vi "Read OD data.vi"(4 "OD num":dbl) -> (1 "OD data":dbl[][](array[numeric]) caption="所有行" format="%0.3f")   [LabVIEW 2013]
panel:
  out "路径":path
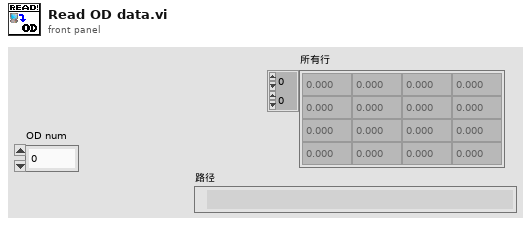
[diagram p1: front panel]
types:
  T1 = typedef "imagedata.ctl" = cluster{"image type":i32, "image depth":i32, "image":u8[], "mask":u8[], "colors":u32[], "Rectangle":cluster{"left":i16, "top":i16, "right":i16, "bottom":i16}}
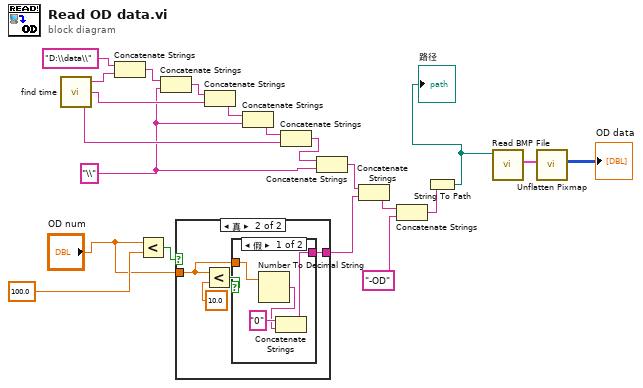
[diagram p0: block diagram]
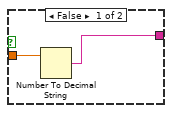
[diagram p2: hidden frame]
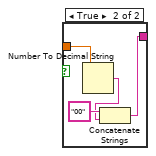
[diagram p3: hidden frame]
diagram:
  w12 = "\\" ("字符串")
  n1 = call "find time.vi"() -> ("day"=w14:string, "month"=w17:string, "year"=w20:string)  [unwired: 3 in]
  n2 = Concatenate Strings("D:\\data\\", w20) -> (w19:string)
  n3 = Less?(x="OD num", y=100.0) -> (x < y?=w6:bool)
  n4 = Concatenate Strings(w19, w12) -> (w18:string)
  n5 = case shown="真" w6 {
    tunnel: "OD num" -> [w23 w25]
    tunnel: [w22 w24] -> w4
    frame False {
      n6 = Number To Decimal String(number=w23) -> (decimal integer string=w22:string)  [unwired: 1 in]
    }
    frame True {
      n7 = Less?(x=w25, y=10.0) -> (x < y?=w26:bool)
      n8 = case shown="假" w26 {
        tunnel: w25 -> [w30 w35]
        tunnel: [w28 w32] -> w24
        frame False {
          n9 = Number To Decimal String(number=w30) -> (decimal integer string=w29:string)  [unwired: 1 in]
          n10 = Concatenate Strings("0" ("字符串"), w29) -> (w28:string)
        }
        frame True {
          n11 = Number To Decimal String(number=w35) -> (decimal integer string=w33:string)  [unwired: 1 in]
          n12 = Concatenate Strings("00" ("字符串"), w33) -> (w32:string)
        }
      }
    }
  }
  n13 = Concatenate Strings(w18, w17) -> (w16:string)
  n14 = Concatenate Strings(w16, w12) -> (w15:string)
  n15 = Concatenate Strings(w15, w14) -> (w13:string)
  n16 = Concatenate Strings(w13, w12) -> (w11:string)
  n17 = Concatenate Strings(w11, w4) -> (w10:string)
  n18 = Concatenate Strings(w10, "-OD" ("字符串")) -> (w8:string)
  n19 = String To Path(string=w8) -> (path=w3:path)
  "路径" <- w3
  n20 = call <vilib>:"Read BMP File.vi"("path to BMP file"=w3) -> ("image data"=w2:T1)  [unwired: 8 in, 2 out]
  n21 = call <vilib>:"Unflatten Pixmap.vi"("image data"=w2) -> ("8-bit pixmap"=→"OD data":u8[][])  [unwired: 4 in, 6 out]
